vi "Sync.Stop.vi"(8 "error in (no error)":errorcluster, 11 "DAQmx in":refnum<class "DAQmx.lvclass">) -> (0 "error out":errorcluster, 3 "DAQmx out":refnum<class "DAQmx.lvclass">)   [LabVIEW 2019, in "DAQmx.lvclass"]
uses:
  DAQmx.lvclass
  DAQmx.lvclass/DAQmx.ctl
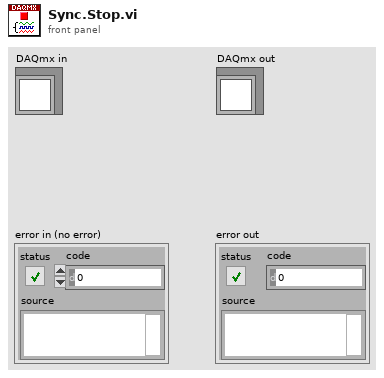
[diagram p1: front panel]
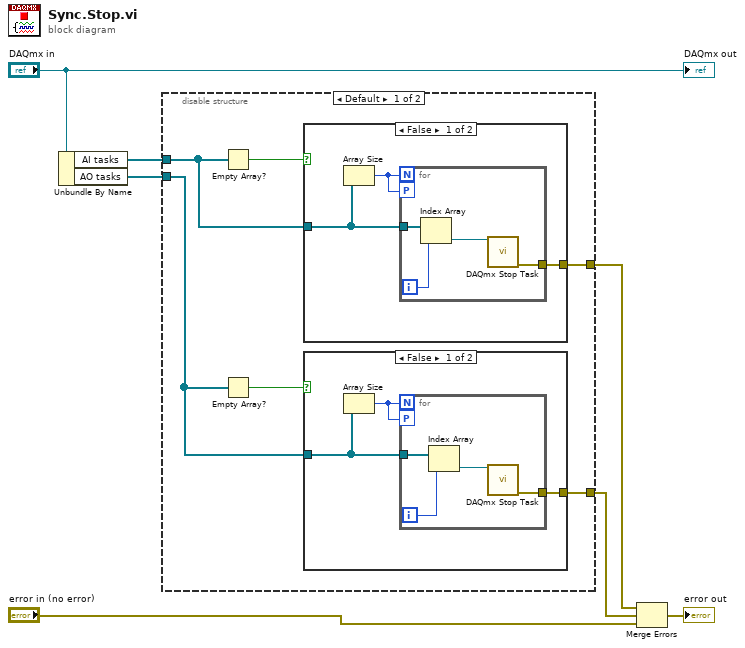
[diagram p0: block diagram]
diagram:
  n1 = Unbundle By Name("DAQmx in") -> ("AI tasks"=w6:refnum<k21>[], "AO tasks"=w7:refnum<k21>[])
  n2 = disable-structure shown="Default" {
    disable-tunnel: [w13 _] -> w3
    disable-tunnel: w7 -> [w9 _]
    disable-tunnel: w6 -> [w11 _]
    disable-tunnel: [w8 _] -> w1
    frame condition #0 (active) {
      n3 = Empty Array?(array=w11) -> (empty?=w12:bool)
      n4 = Empty Array?(array=w9) -> (empty?=w10:bool)
      n5 = case shown="False" w12 {
        tunnel: w11 -> [w22 _]
        tunnel: [w23 _] -> w13
        frame False {
          n6 = Array Size(array=w22) -> (size(s)=w21:i32)
          n7 = for {
            N: w21 -> [_]
            tunnel: w22 -> [w26]
            tunnel: [w27] -> w23
            workers-P: w21 -> [_]
            i -> [w25]
            n8 = Index Array(array=w26, index=w25) -> (element=w24:refnum<k21>)
            n9 = call <vilib>:"DAQmx Stop Task.vi"("task/channels in"=w24) -> ("error out"=w27:errorcluster)  [unwired: 13 in, 1 out]
          }
        }
        frame True {
        }
      }
      n10 = case shown="False" w10 {
        tunnel: w9 -> [w15 _]
        tunnel: [w16 _] -> w8
        frame False {
          n11 = Array Size(array=w15) -> (size(s)=w14:i32)
          n12 = for {
            N: w14 -> [_]
            tunnel: w15 -> [w19]
            tunnel: [w20] -> w16
            workers-P: w14 -> [_]
            i -> [w18]
            n13 = Index Array(array=w19, index=w18) -> (element=w17:refnum<k21>)
            n14 = call <vilib>:"DAQmx Stop Task.vi"("task/channels in"=w17) -> ("error out"=w20:errorcluster)  [unwired: 13 in, 1 out]
          }
        }
        frame True {
        }
      }
    }
    frame condition #1 {
    }
  }
  n15 = Merge Errors(w3, w1, "error in (no error)") -> (→"error out":errorcluster)
  "DAQmx out" <- "DAQmx in"
